vi "Sort 2D String Array - Generate Format String.vi"(5 "Input String (\" \")":string, 9 "Number":dbl format="%.12f") -> (6 "Format String":string, 10 "Number Out":dbl format="%.12f")   [LabVIEW 2009, in "xijk_select_best_filter.lvlib"]
doc: "Sort 2D String Array - Generate Format String.vi\n\n<B>Description:</B>\n\nThis VI Generates a string representing the numeric format of the input string.\n\n\n<B>Usage:</B>\n\nWire all required inputs.\n\n<B>Inputs:</B>\n\nNumber\n- This is the input string represented as a number.\n\nInput String\n- This is the string that the VI generates a format string for.\n\n<B>Outputs:</B>\n\nNumber Out\n- This is Number passed to Number Out.\n\nFormat String\n- This is the format string that the VI generated for the input string.\n\n<B>Developed by:</B>\n\nMark Ridgley\nmark.ridgley@logicpd.com"
uses:
  xijk_select_best_filter.lvlib
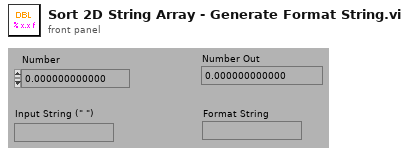
[diagram p1: front panel]
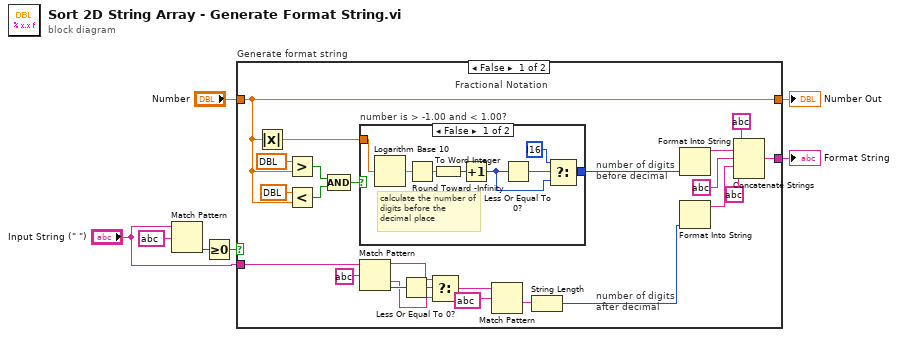
[diagram p0: block diagram]
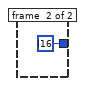
[diagram p2: hidden frame]
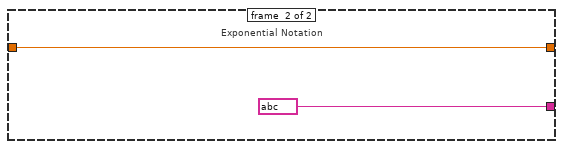
[diagram p3: hidden frame]
diagram:
  n1 = Match Pattern(string="Input String (\" \")", regular expression=string ?) -> (offset past match=w4:i32)  [unwired: 4 out]
  n2 = Greater Or Equal To 0?(x=w4) -> (x >= 0?=w3:bool)
  n3 = case "Generate format string" shown="False" w3 {
    tunnel: [w31 string ?] -> w7
    tunnel: "Input String (\" \")" -> [w11 _]
    tunnel: "Number" -> [w13 w41]
    tunnel: [w13 w41] -> w1
    frame #0 {
      # "number of digits after decimal"
      # "Fractional Notation"
      # "number of digits before decimal"
      n4 = Absolute Value(x=w13) -> (abs(x)=w26:dbl)
      n5 = Greater?(x=dbl ?, y=w13) -> (0:w16:bool)
      n6 = Less?(x=dbl ?, y=w13) -> (x < y?=w15:bool)
      n7 = Compound Arithmetic op=AND(w16, w15) -> (w14:bool)
      n8 = case "number is > -1.00 and < 1.00?" shown="False" w14 {
        tunnel: [w35 i16 ?] -> w24
        tunnel: w26 -> [w36 _]
        frame #0 {
          # "calculate the number of digits before the decimal place"
          n9 = Logarithm Base 10(1:w36) -> (0:w39:dbl)
          n10 = Round Toward -Infinity(1:w39) -> (0:w38:dbl)
          n11 = To Word Integer(number=w38) -> (16bit integer=w37:i16)
          n12 = Increment(x=w37) -> (x+1=w34:i16)
          n13 = Less Or Equal To 0?(x=w34) -> (x <= 0?=w32:bool)
          n14 = Select(t=i16 ?, s=w32, f=w34) -> (s? t:f=w35:i16)
        }
        frame #1 {
        }
      }
      n15 = Match Pattern(string=w11, regular expression=string ? ("search char (-)")) -> (before substring=w20:string, after substring=w12:string, offset past match=w21:i32)  [unwired: 2 out]
      n16 = Less Or Equal To 0?(x=w21) -> (x <= 0?=w22:bool)
      n17 = Select(t=w20, s=w22, f=w12) -> (s? t:f=w10:string)
      n18 = Match Pattern(string=w10, regular expression=string ?) -> (after substring=w9:string)  [unwired: 4 out]
      n19 = String Length(string=w9) -> (length=w8:i32)
      n20 = Format Into String(w24) -> (resulting string=w29:string)  [unwired: 3 in, 1 out]
      n21 = Format Into String(w8) -> (resulting string=w27:string)  [unwired: 3 in, 1 out]
      n22 = Concatenate Strings(string ? ("Substring"), w29, string ? ("Substring"), w27, string ?) -> (w31:string)
    }
    frame #1 {
      # "Exponential Notation"
    }
  }
  "Format String" <- w7
  "Number Out" <- w1
